vi "Replace Tag with Array.vi"(8 "Error In":errorcluster caption="Error in (no error)", 9 "Tag":enum16{"<1>", "<2>", "<3>", "<4>"}(ring), 10 "Replace String":string[](array[string]), 11 "Single-line Text":string="All Data Saved@TDMS >> API: Terminate@<1> -><register>") -> (0 "Error Out":errorcluster, 3 "States":string)   [LabVIEW 2017, in "Communicable State Machine.lvlib"]
doc: "### Replace Tag with Array.vi\n\n-- <b>Controls</b> --\n- <b>Enum</b>:\n- <b>replace string</b>:\n- <b>single-line text</b>:\n\n-- <b>Indicators</b> --\n- <b>States</b>:"
uses:
  Communicable State Machine.lvlib
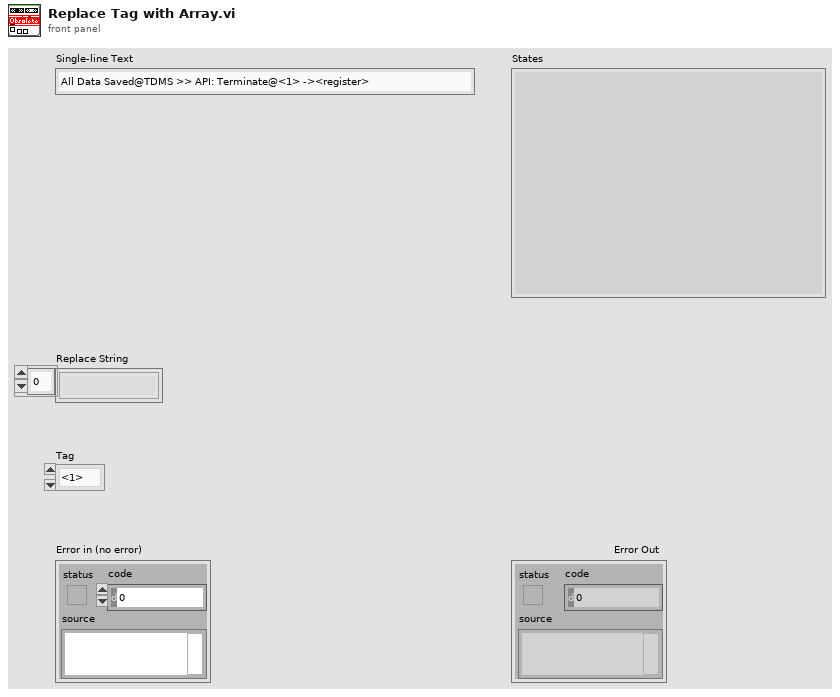
[diagram p1: front panel]
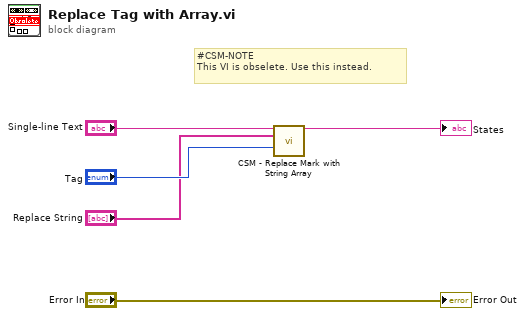
[diagram p0: block diagram]
diagram:
  # "#CSM-NOTE\nThis VI is obselete. Use this instead."
  n1 = call "CSM - Replace Mark with String Array.vi"("Single-line Text"="Single-line Text", "Replace String"="Replace String", "Substitution Mark"="Tag") -> ("States"=→"States":string)  [unwired: 12 in]
  "Error Out" <- "Error In"
